vi "Set Data Type.vi"(8 "error in":errorcluster, 10 "Data Type":T1=1 items=["unknown", "BOOLEAN", "INTEGER8", "INTEGER16", "INTEGER32", "UNSIGNED8", "UNSIGNED16", "UNSIGNED32", "REAL32", "VISIBLE_STRING", "OCTET_STRING", "UNICODE_STRING", "TIME_OF_DAY", "TIME_DIFFERENCE", "RESERVED1", "DOMAIN", "INTEGER24", "REAL64", "INTEGER40", "INTEGER48", "INTEGER56", "INTEGER64", "UNSIGNED24", "RESERVED2", "UNSIGNED40", "UNSIGNED48", "UNSIGNED56", "UNSIGNED64", "RESERVED3", "RESERVED4", "RESERVED5", "RESERVED6", "PDO_COMMUNICATION_PARAMETER", "PDO_MAPPING", "SDO_PARAMETER", "IDENTITY", "RESERVED7"], 11 "Object Entry in":refnum<class "Object Entry.lvclass">) -> (0 "error out":errorcluster, 3 "Object Entry out":refnum<class "Object Entry.lvclass">)   [LabVIEW 2020, in "CANopen.lvlib" / "Object Entry.lvclass"]
uses:
  Object Entry.lvclass
  Object Entry.lvclass/Object Entry.ctl
  Sub Object/Sub Object.lvclass
  Typedefs/Data Type.ctl
  CANopen.lvlib
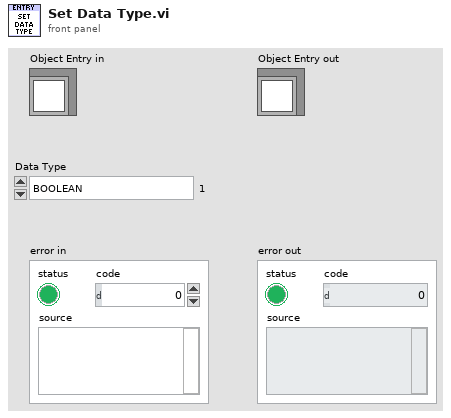
[diagram p1: front panel]
types:
  T1 = typedef "CANopen.lvlib/Data Type.ctl" = u16
  T2 = typedef "CANopen.lvlib/Object Type.ctl" = u8
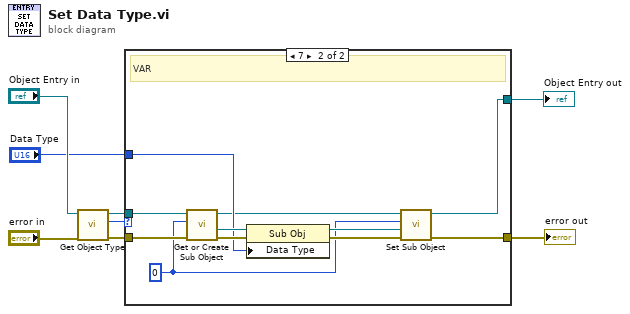
[diagram p0: block diagram]
diagram:
  n1 = call "Get Object Type.vi"("error in"="error in", "Object Entry in"="Object Entry in") -> ("error out"=w6:errorcluster, "Object Type"=w7:T2, "Object Entry out"=w8:refnum<class "Object Entry.lvclass">)  [unwired: 7 in]
  n2 = case shown="7" w7 {
    tunnel: [w9 w13] -> w1
    tunnel: "Data Type" -> [_ w16]
    tunnel: w8 -> [w9 w19]
    tunnel: w6 -> [w10 w21]
    tunnel: [w10 w15] -> w4
    frame Default {
    }
    frame 7 {
      w11 = u8 0 ("Sub Index")
      # "VAR"
      n3 = call "Get or Create Sub Object.vi"("error in"=w21, "Sub Index"=w11, "Obj Entry in"=w19) -> ("error out"=w20:errorcluster, "Sub Object"=w17:refnum<class "Sub Object.lvclass">, "Obj Entry out"=w14:refnum<class "Object Entry.lvclass">)  [unwired: 6 in]
      n4 = property class="Sub Obj"(reference=w17, error in=w20, "Data Type"=w16) -> (reference out=w12:refnum<class "Sub Object.lvclass">, error out=w18:errorcluster)
      n5 = call "Set Sub Object.vi"("error in"=w18, "Sub Object"=w12, "Sub Index"=w11, "Obj Entry in"=w14) -> ("error out"=w15:errorcluster, "Obj Entry out"=w13:refnum<class "Object Entry.lvclass">)  [unwired: 6 in]
    }
  }
  "error out" <- w4
  "Object Entry out" <- w1
